vi "Sleep.vi"(8 "error in (no error)":errorcluster, 11 "CIFCorePlugin in":refnum<class "CIFCorePlugin.lvclass">) -> (0 "error out":errorcluster, 2 "Housekeep only":bool, 3 "CIFCorePlugin out":refnum<class "CIFCorePlugin.lvclass">)   [LabVIEW 2021, in "CIFCorePlugin.lvclass"]
uses:
  CIFCorePlugin.lvclass
  CIFCorePlugin.lvclass/CIFCorePlugin.ctl
  Common/Typedef/Errors.ctl
  Accessors/Read Sleep Limits (ns).vi
  Accessors/Timestamps/Write Target Wake TS.vi
  Accessors/Timestamps/Read Running TS.vi
  Accessors/Read Running Internal Data.vi
  Accessors/Read Timing Override.vi
  Accessors/Read Common Config.vi
  <vilib>/CIF Foundation/CIF Utilities/Time/System Time/LabVIEW Time to TAI Time.vi
  <vilib>/CIF Foundation/CIF Utilities/Errors/Append Error Location.vi
  Common/CIFCoreCommon.lvlib
  <vilib>/CIF Foundation/CIF Utilities/Time/Time_CIF_U.lvlib
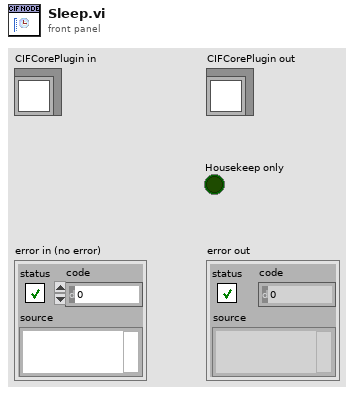
[diagram p1: front panel]
types:
  T1 = typedef "CIFCoreCommon.lvlib/Errors.ctl" = enum16{"Invalid Clock ID", "Long Sleep", "gRPC Server Not Found", "Config Parse", "Timestamp Wrap", "Delayed Execution", "Duplicate Channel", "Missing Channel", "Incorrect Type", "Flatten Error", "Unflatten Data", "Unique Name", "Plugin Not Found", "Plugin Type Not Found", "Plugin Version Not Found", "Manager Not Found", "Numerical Issue", "Time Jump", "Clock ID Match", "Channel Length", "Plugin Connection", "gRPC Server Connection", "PPL Name Match", "Build", "Config Log Parse", "Plugin Load", "UI Subpanel Load", "Python Name", "Invalid Name", "Unable to Change Ch Buffer"}
  T2 = typedef "CIFCoreCommon.lvlib/Timing Overrides.ctl" = cluster{"Override Timing":bool, "Skip Sleep":bool, "Period (s)":dbl}
  T3 = typedef "CIFCorePlugin.lvclass/Running Internal Data.ctl" = cluster{"Refresh":bool, "Iterations":i64, "Housekeep only":bool, "Configured period (ns)":i64, "Update channel OOB":bool, "Configuration Change":bool, "Disable Auto Benchmark":bool, "gRPC Loop":bool}
  T4 = typedef "CIFCoreCommon.lvlib/Common Plugin Configuration.ctl" = cluster{"Period (s)":dbl, "Offset (us)":i32, "Priority":i32, "Processor":i32, "External Clock":T5}
  T5 = typedef "CIFCoreCommon.lvlib/External Clock Config.ctl" = cluster{"ClockID":u8, "Clock Name":string, "Clock Source":bool, "Convert Data Timestamps":bool, "Use for Timing":bool}
  T6 = typedef "Time_CIF_U.lvlib/Future Time Event Limits.ctl" = cluster{"Maximum":i64, "Minimum":i64}
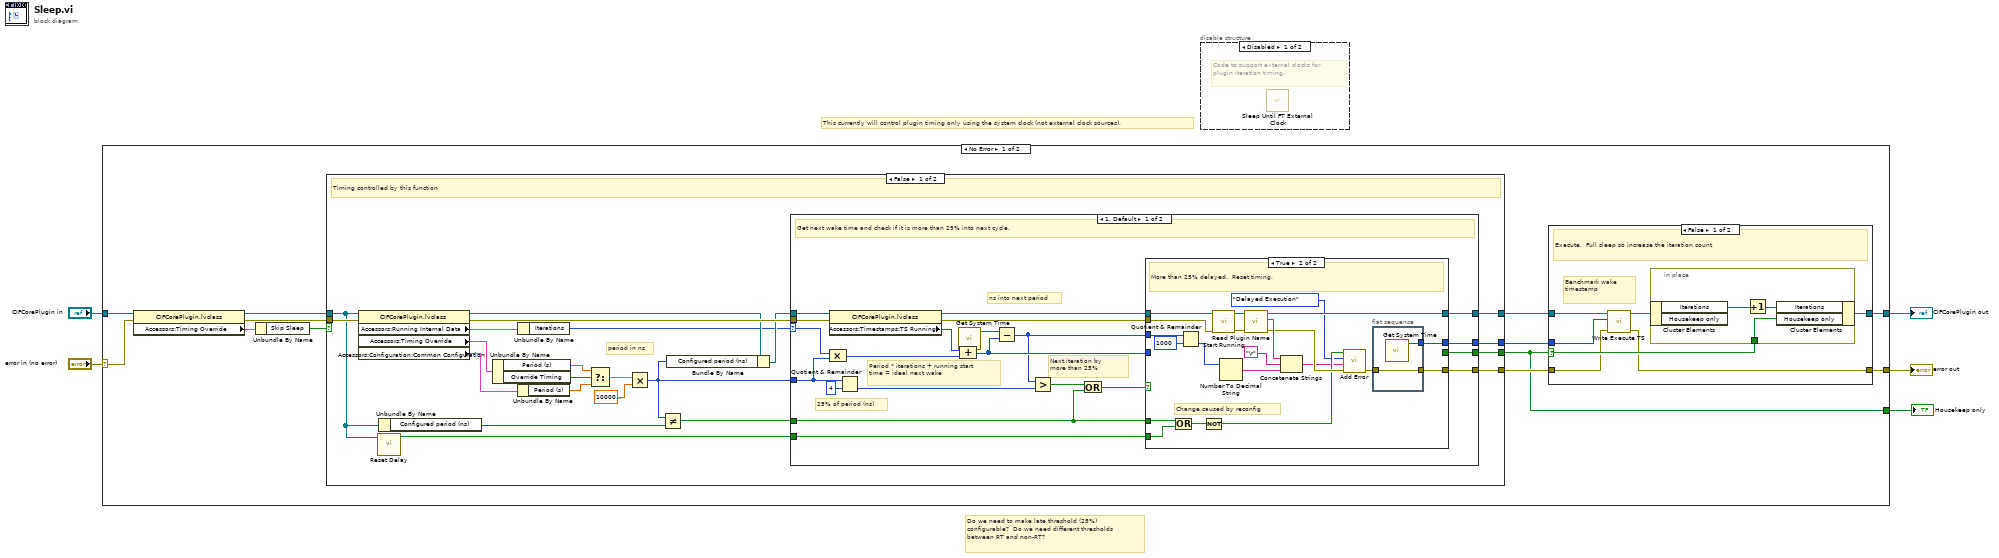
[diagram p0: block diagram]
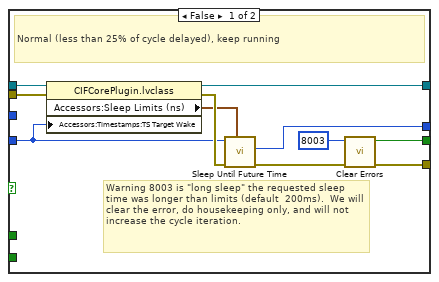
[diagram p3: hidden frame]
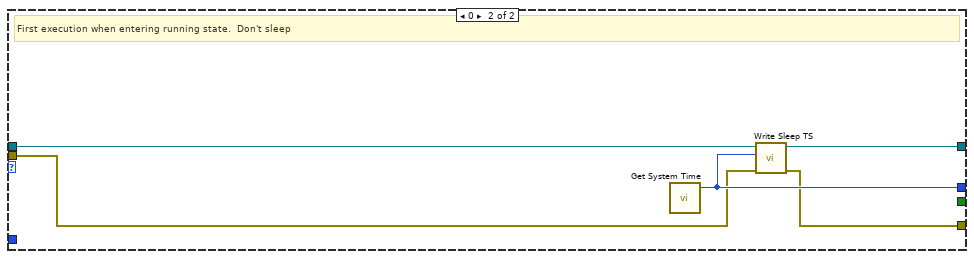
[diagram p4: hidden frame]
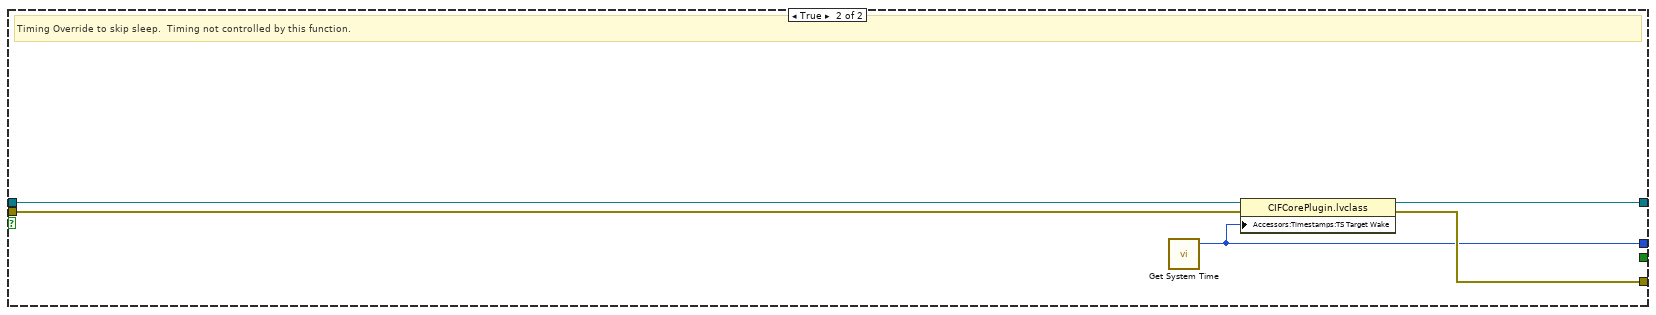
[diagram p5: hidden frame]
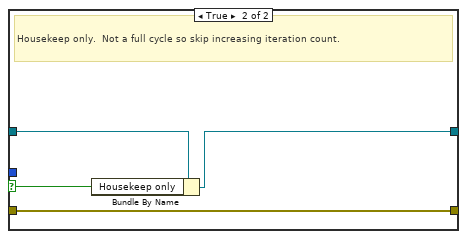
[diagram p6: hidden frame]
diagram:
  # "This currently will control plugin timing only using the system clock (not external clock sources)."
  # "Do we need to make late threshold (25%) configurable?  Do we need different thresholds between RT and non-RT?"
  n1 = case shown="No Error" "error in (no error)" {
    selector: "error in (no error)" -> [w11 w120]
    tunnel: [w13 w120] -> w1
    tunnel: [w16 w119] -> w3
    tunnel: "CIFCorePlugin in" -> [w12 w119]
    tunnel: [w6 _] -> w2
    frame No Error {
      n2 = property class="CIFCorePlugin.lvclass"(reference=w12, error in=w11) -> (reference out=w10:refnum<class "CIFCorePlugin.lvclass">, error out=w9:errorcluster, "Accessors:Timing Override"=w8:T2)
      n3 = Unbundle By Name(w8) -> ("Skip Sleep"=w7:bool)
      n4 = case shown="False" w7 {
        tunnel: [w39 w104] -> w17
        tunnel: [w25 _] -> w6
        tunnel: [w22 w101] -> w15
        tunnel: [w21 w102] -> w14
        tunnel: w10 -> [w19 w100]
        tunnel: w9 -> [w20 w103]
        frame False {
          # "period in ns"
          # "Timing controlled by this function"
          n5 = property class="CIFCorePlugin.lvclass"(reference=w19, error in=w20) -> (reference out=w28:refnum<class "CIFCorePlugin.lvclass">, error out=w38:errorcluster, "Accessors:Running Internal Data"=w24:T3, "Accessors:Timing Override"=w30:T2, "Accessors:Configuration:Common Configuration"=w33:T4)
          n6 = call "Reset Delay.vi"("CIFCorePlugin in"=w19) -> ("Reset"=w18:bool)  [unwired: 3 in]
          n7 = Unbundle By Name(w19) -> ("Configured period (ns)"=w29:i64)
          n8 = Unbundle By Name(w30) -> ("Period (s)"=w32:dbl, "Override Timing"=w34:bool)
          n9 = Unbundle By Name(w33) -> ("Period (s)"=w37:dbl)
          n10 = Unbundle By Name(w24) -> ("Iterations"=w23:i64)
          n11 = Select(t=w32, s=w34, f=w37) -> (s? t:f=w35:dbl)
          n12 = Multiply(x=w35, y=1000000000.0 ("x")) -> (x*y=w26:i64)
          n13 = Not Equal?(x=w26, y=w29) -> (x != y?=w31:bool)
          n14 = Bundle By Name(cluster=w28, "Configured period (ns)"=w26) -> (w27:refnum<class "CIFCorePlugin.lvclass">)
          n15 = case shown="1, Default" w23 {
            selector: w23 -> [w45 _]
            tunnel: [w59 w98] -> w39
            tunnel: w38 -> [w60 w96]
            tunnel: w27 -> [w52 w99]
            tunnel: [w58 w95] -> w21
            tunnel: w26 -> [w43 _]
            tunnel: w31 -> [w55 _]
            tunnel: [w54 _] -> w25
            tunnel: [w53 w97] -> w22
            tunnel: w18 -> [w40 _]
            frame 1, Default {
              # "ns into next period"
              # "25% of period (ns)"
              # "Next iteration by more than 25%"
              # "Period * iterations + running start time = ideal next wake"
              # "Get next wake time and check if it is more than 25% into next cycle."
              n16 = property class="CIFCorePlugin.lvclass"(reference=w52, error in=w60) -> (reference out=w42:refnum<class "CIFCorePlugin.lvclass">, error out=w57:errorcluster, "Accessors:Timestamps:TS Running"=w51:i64)
              n17 = Compound Arithmetic op=MULTIPLY(w45, w43) -> (w50:i64)
              n18 = Quotient & Remainder(x=w43, y=i64 4) -> (floor(x/y)=w44:i64)  [unwired: 1 out]
              n19 = call <vilib>:"Get System Time.vi"() -> ("Time (ns)"=w49:i64)  [unwired: 5 in]
              n20 = Compound Arithmetic op=ADD(w51, w50) -> (w48:i64)
              n21 = Subtract(x=w49, y=w48) -> (x-y=w41:i64)
              n22 = Greater?(x=w41, y=w44) -> (0:w47:bool)
              n23 = Compound Arithmetic op=OR(w47, w55) -> (w56:bool)
              n24 = case shown="True" w56 {
                tunnel: w42 -> [w63 w92]
                tunnel: [w61 w90] -> w59
                tunnel: w57 -> [w71 w91]
                tunnel: [w70 w86] -> w58
                tunnel: w55 -> [_ w79]
                tunnel: w48 -> [w65 _]
                tunnel: [w68 _] -> w54
                tunnel: [w64 w87] -> w53
                tunnel: w41 -> [_ w85]
                tunnel: w40 -> [_ w78]
                frame False {
                  # "Warning 8003 is \"long sleep\" the requested sleep time was longer than limits (default  200ms).  We will clear the error, do housekeeping only, and will not increase the cycle iteration."
                  # "Normal (less than 25% of cycle delayed), keep running"
                  n25 = property class="CIFCorePlugin.lvclass"(reference=w63, error in=w71, "Accessors:Timestamps:TS Target Wake"=w65) -> (reference out=w61:refnum<class "CIFCorePlugin.lvclass">, error out=w67:errorcluster, "Accessors:Sleep Limits (ns)"=w62:T6)
                  n26 = call <vilib>:"Sleep Until Future Time.vi"("FTE Limits (ns)"=w62, "error in (no error)"=w67, "Wake Time (ns)"=w65) -> ("error out"=w66:errorcluster, "Wake Time (ns)"=w64:i64)  [unwired: 6 in, 1 out]
                  n27 = call <vilib>:"Clear Errors.vi"("error in (no error)"=w66, "specific error code to clear (0: all)"=8003 ("code")) -> ("error out"=w70:errorcluster, "specific error cleared?"=w68:bool)  [unwired: 4 in]
                }
                frame True {
                  # "Change caused by reconfig"
                  # "More than 25% delayed.  Reset timing."
                  n28 = Compound Arithmetic op=OR(w79, w78) -> (w77:bool)
                  n29 = Quotient & Remainder(x=w85, y=i64 1000) -> (floor(x/y)=w83:i64)  [unwired: 1 out]
                  n30 = Not(x=w77) -> (.not. x?=w74:bool)
                  n31 = call "Start Running.vi"("error in (no error)"=w91, "CIFCorePlugin in"=w92) -> ("error out"=w88:errorcluster, "CIFCorePlugin out"=w89:refnum<class "CIFCorePlugin.lvclass">)  [unwired: 8 in]
                  n32 = Number To Decimal String(number=w83) -> (decimal integer string=w81:string)  [unwired: 1 in]
                  n33 = call "Read Plugin Name.vi"("error in (no error)"=w88, "CIFTemplateNode in"=w89) -> ("error out"=w76:errorcluster, "Plugin Name"=w82:string, "CIFTemplateNode out"=w90:refnum<class "CIFCorePlugin.lvclass">)  [unwired: 7 in]
                  n34 = Concatenate Strings(w82, "\r", w81) -> (w72:string)
                  n35 = call <vilib>:"Add Error.vi"("error in (no error)"=w76, "String to Append"=w72, "Error"=Errors."Delayed Execution", "Insert Error"=w74) -> ("error out"=w75:errorcluster)  [unwired: 7 in]
                  n36 = flat-sequence {
                    tunnel: [w94] -> w87
                    tunnel: w75 -> [w93]
                    tunnel: [w93] -> w86
                    frame #0 {
                      n37 = call <vilib>:"Get System Time.vi"() -> ("Time (ns)"=w94:i64)  [unwired: 5 in]
                    }
                  }
                }
              }
            }
            frame 0 {
              # "First execution when entering running state.  Don't sleep"
              n38 = call <vilib>:"Get System Time.vi"() -> ("Time (ns)"=w97:i64)  [unwired: 5 in]
              n39 = call "Write Sleep TS.vi"("error in (no error)"=w96, "Sleep"=w97, "CIFCorePlugin in"=w99) -> ("error out"=w95:errorcluster, "CIFCorePlugin out"=w98:refnum<class "CIFCorePlugin.lvclass">)  [unwired: 7 in]
            }
          }
        }
        frame True {
          # "Timing Override to skip sleep.  Timing not controlled by this function."
          n40 = call <vilib>:"Get System Time.vi"() -> ("Time (ns)"=w101:i64)  [unwired: 5 in]
          n41 = property class="CIFCorePlugin.lvclass"(reference=w100, error in=w103, "Accessors:Timestamps:TS Target Wake"=w101) -> (reference out=w104:refnum<class "CIFCorePlugin.lvclass">, error out=w102:errorcluster)
        }
      }
      n42 = case shown="False" w6 {
        selector: w6 -> [w110 w116]
        tunnel: w17 -> [w106 w118]
        tunnel: [w111 w117] -> w16
        tunnel: w15 -> [w107 _]
        tunnel: w14 -> [w105 w115]
        tunnel: [w108 w115] -> w13
        frame False {
          # "Benchmark wake timestamp"
          # "Execute.  Full sleep so increase the iteration count"
          n43 = call "Write Execute TS.vi"("error in (no error)"=w105, "Execute"=w107, "CIFCorePlugin in"=w106) -> ("error out"=w108:errorcluster, "CIFCorePlugin out"=w109:refnum<class "CIFCorePlugin.lvclass">)  [unwired: 7 in]
          n44 = in-place {
            in-place-border: w110 -> [w114]
            n45 = in-place-cluster #1(w109) -> ("Iterations"=w113:i64)  [unwired: 1 out]
            n46 = Increment(x=w113) -> (x+1=w112:i64)
            n47 = in-place-cluster #1("Iterations"=w112, "Housekeep only"=w114) -> (w111:refnum<class "CIFCorePlugin.lvclass">)
          }
        }
        frame True {
          # "Housekeep only.  Not a full cycle so skip increasing iteration count."
          n48 = Bundle By Name(cluster=w118, "Housekeep only"=w116) -> (w117:refnum<class "CIFCorePlugin.lvclass">)
        }
      }
    }
    frame Error {
    }
  }
  "error out" <- w1
  "CIFCorePlugin out" <- w3
  "Housekeep only" <- w2
  n49 = disable-structure shown="Disabled" {
    frame Disabled {
      # "Code to support external clocks for plugin iteration timing."
      n50 = call "Sleep Until FT External Clock.vi"() -> ()  [unwired: 8 in, 4 out]
    }
    frame Enabled {
    }
  }
